vi "Red_INI_Value.vi"(10 "section":string, 11 "section 2":string) -> (3 "value":string)   [LabVIEW 2018]
uses:
  Subvi/Global.vi
  <vilib>/Utility/config.llb/Read Key (String).vi
  <vilib>/Utility/config.llb/NI_LVConfig.lvlib
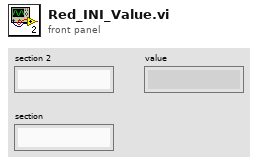
[diagram p1: front panel]
types:
  T1 = typedef "NI_LVConfig.lvlib/Config Data RefNum.ctl" = refnum<k1>
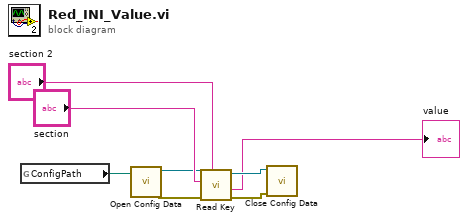
[diagram p0: block diagram]
diagram:
  n1 = global read "Global.vi" "ConfigPath"() -> (w1:path)
  n2 = call <vilib>:"Open Config Data.vi"("configuration file path"=w1) -> ("error out"=w8:errorcluster, "refnum"=w3:T1)  [unwired: 8 in, 1 out]
  n3 = call-poly <vilib>:"Read Key.vi"("section"="section 2", "error in (no error)"=w8, "key"="section", "refnum"=w3) -> ("error out"=w7:errorcluster, "value"=→"value":string, "refnum out"=w6:T1)  [unwired: 4 in, 1 out]
  n4 = call <vilib>:"Close Config Data.vi"("error in (no error)"=w7, "refnum"=w6) -> ()  [unwired: 8 in, 2 out]
